vi "MODBUS  SLAVE.vi"() -> (3 "values to write":u16[](array[numeric]) caption="待写入值")   [LabVIEW 2016]
uses:
  <vilib>/NI/Modbus Library/Data Model/Device Data Model.lvclass
  <vilib>/NI/Modbus Library/API/Wrapper/Create TCP Slave.vi
  <vilib>/NI/Modbus Library/API/Slave/Modbus Slave.lvclass
  <vilib>/NI/Modbus Library/API/Wrapper/API Main.lvlib
panel:
  out "运行周期":u16[](array[numeric])
  in  "write operation starting address":u16=100 caption="写操作起始地址"
  out "单仪器启动命令":u16[](array[numeric])
  out "系统启动命令":u16[](array[numeric])
  in  "停止":bool
  out "register values":u16[](array[numeric]) caption="寄存器值"
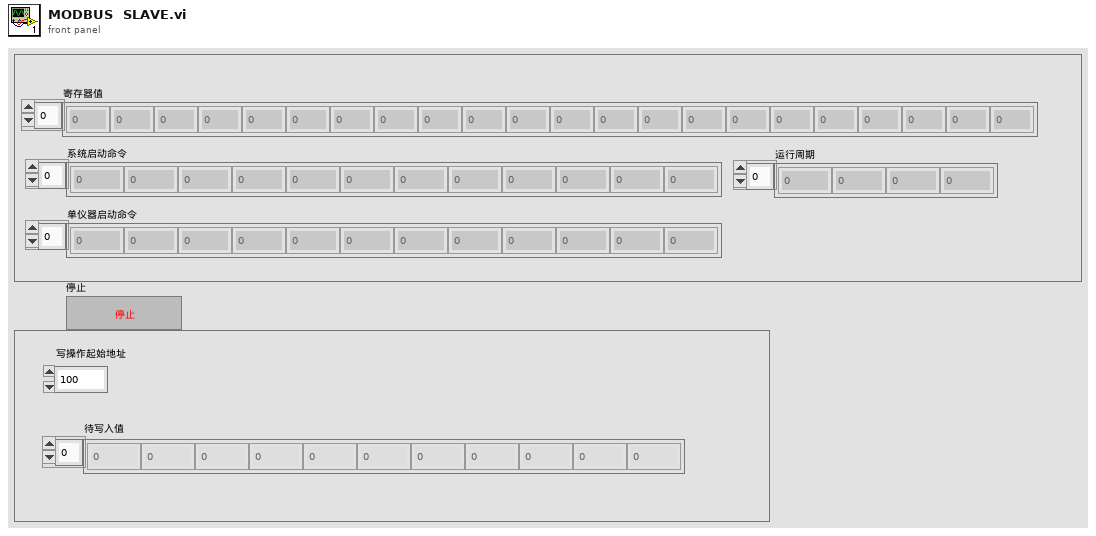
[diagram p1: front panel]
types:
  T1 = cluster{"测量模式":enum16{"水样测量", "标样核查", "零点核查", "跨度核查", "空白测试", "加标回收", "平行样", "校零", "校标"}}
  T2 = cluster{"站号":u16, "量程切换":enum32{"H", "L", "AUTO"}, "控制命令":enum16{"启动测量", "标样核查", "零点核查", "跨度核查", "空白测试", "平行样测试", "加标回收", "空白校准", "标样校准", "初始化（清洗）", "停止测试", "仪器重启", "校时", "模式设置", "测量间隔设置"}, "模式设置":enum16{"待机", "连续模式", "周期模式", "定点模式", "受控模式", "手动模式"}, "测量间隔":u16}
  T3 = cluster{"系统时间":timestamp, "工作状态":enum16{"空闲", "水样测试", "标样核查", "零点核查", "跨度核查", "空白测试", "平行样测试", "加标回收", "空白校准", "标样校准", "初始化（清洗）"}, "测量模式":enum16{"待机", "连续模式", "周期模式", "定点模式", "受控模式", "手动模式"}, "告警代码":enum16{"无告警", "缺试剂告警", "缺水样告警", "缺蒸馏水告警", "缺标液告警", "仪表漏液告警", "标定异常告警", "超量程告警", "加热异常", "低试剂预警", "超上限告警", "超下限告警", "仪表内部其他异常", "滴定异常告警", "电极异常告警", "量程切换告警", "参数设置告警", "PH电极电位异常", "电导率电极异常", "浊度光度异常", "溶解氧电极异常", "溶解氧光强异常", "温度异常告警", "PH异常告警", "溶解氧异常告警", "电导率异常告警", "浊度异常告警", "叶绿素异常告警", "藻密度异常告警", "蓝绿藻异常告警", "ORP异常告警", "氨氮异常告警", "清洁刷异常告警", "SD卡异常告警", "蓝牙异常告警", "Wifi异常告警", "流程异常告警"}, "故障代码":enum16{"无故障", "电机故障", "温度故障", "通讯故障", "滴定故障"}, "日志代码":u16, "软件版本":u16, "F0":sgl, "F1":sgl, "F2":sgl, "F3":sgl, "T":sgl, "H":sgl, "id":u16, "flowid":u16, "量程":u16, "总磷控温温度1":sgl, "营养盐控温温度2":sgl, "ADC":sgl}
  T4 = enum16{"空闲", "水样测试", "标样核查", "零点核查", "跨度核查", "空白测试", "平行样测试", "质控样", "空白校准", "标样校准", "加标回收"}
  T5 = enum16{"空闲", "水样测试", "标样核查", "零点核查", "跨度核查", "空白测试", "平行样测试", "加标回收", "空白校准", "标样校准", "初始化（清洗）"}
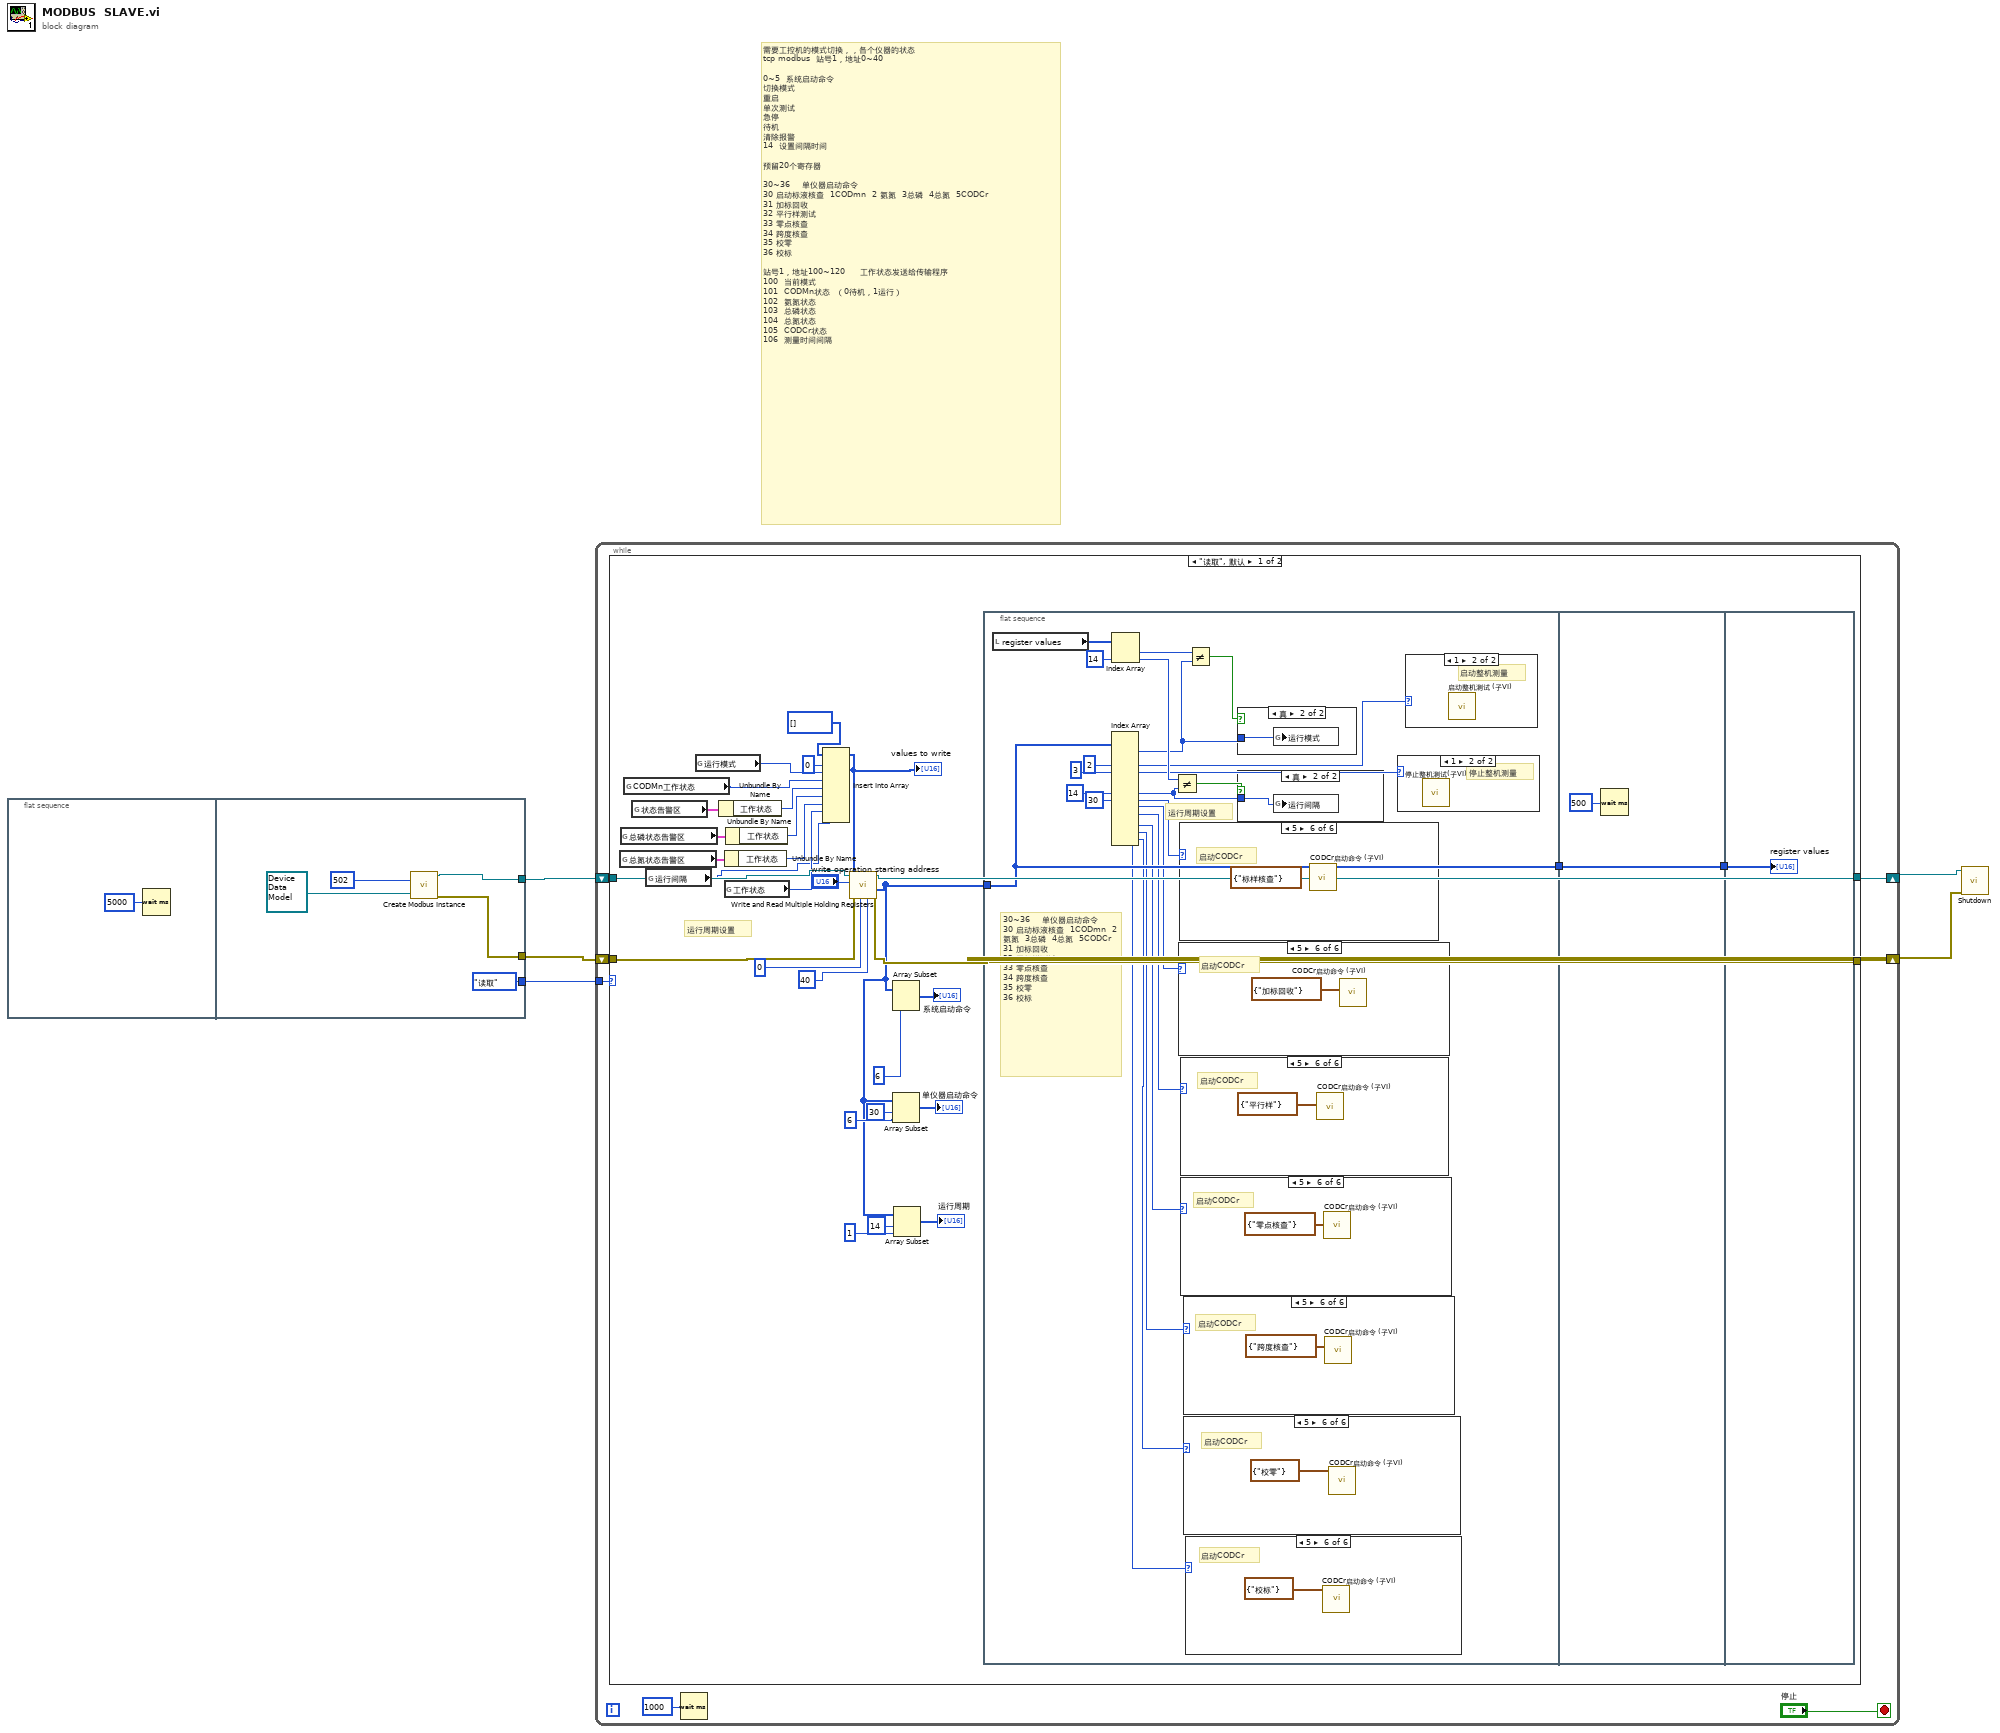
[diagram p0: block diagram]
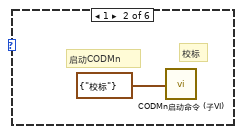
[diagram p3: hidden frame]
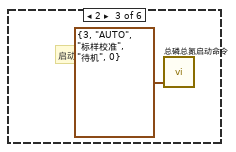
[diagram p4: hidden frame]
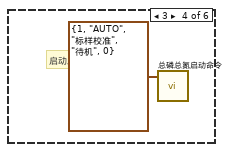
[diagram p5: hidden frame]
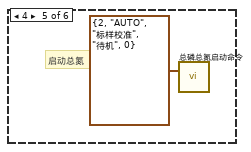
[diagram p6: hidden frame]
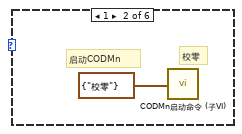
[diagram p8: hidden frame]
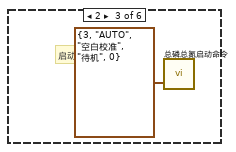
[diagram p9: hidden frame]
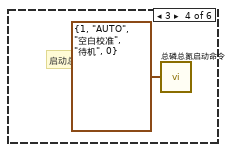
[diagram p10: hidden frame]
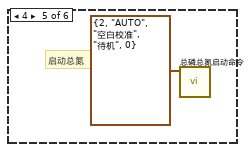
[diagram p11: hidden frame]
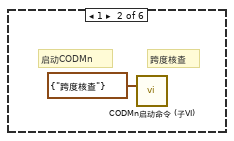
[diagram p13: hidden frame]
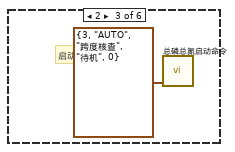
[diagram p14: hidden frame]
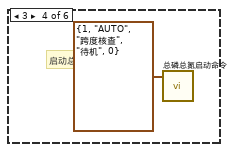
[diagram p15: hidden frame]
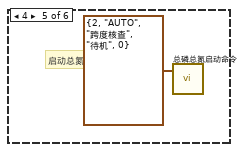
[diagram p16: hidden frame]
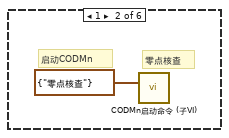
[diagram p18: hidden frame]
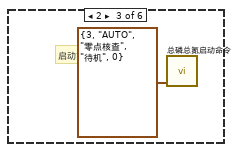
[diagram p19: hidden frame]
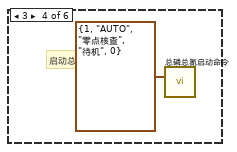
[diagram p20: hidden frame]
diagram:
  # "需要工控机的模式切换，，各个仪器的状态\ntcp modbus  站号1，地址0~40\n\n0~5  系统启动命令\n切换模式\n重启\n单次测试\n急停\n待机\n清除报警\n14  设置间隔时间\n\n预留20个寄存器\n\n30~36    单仪器启动命令\n30 启动标液核查  1CODmn  2 氨氮  3总磷  4总氮  5CODCr\n31 加标回收\n32 平行样测试\n33 零点核查\n34 跨度核查\n35 校零\n36 校标\n\n站号1，地址100~120     工作状态发送给传输程序\n100  当前模式\n101  CODMn状态  （0待机，1运行）\n102  氨氮状态\n103  总磷状态\n104  总氮状态\n105  CODCr状态\n106  测量时间间隔"
  n1 = flat-sequence {
    tunnel: [enum16{"读取", "写入"}."读取"] -> w5
    tunnel: [w9] -> w4
    tunnel: [w8] -> w3
    frame #0 {
      n2 = Wait (ms)(milliseconds to wait=u32 5000 ("等待时间（毫秒）")) -> ()  [unwired: 1 out]
    }
    frame #1 {
      n3 = call-poly <vilib>:"Create Modbus Instance.vi"("device data model"=refnum<class "Device Data Model.lvclass"> refnum, "port (502)"=u16 502) -> ("error out"=w8:errorcluster, "TCP slave instance"=w9:refnum<class "Modbus Slave.lvclass">)  [unwired: 8 in]
    }
  }
  n4 = while {
    shift-right: [w16] -> w2
    shift-left: w4 -> [w18]
    shift-right: [w12] -> w1
    shift-left: w3 -> [w17]
    tunnel: w5 -> [w13]
    stop <- "停止" stop-if-true
    n5 = case shown="\"读取\", 默认" w13 {
      tunnel: w18 -> [w45 w113]
      tunnel: w17 -> [w44 w112]
      tunnel: [w40 w113] -> w16
      tunnel: [w41 w112] -> w12
      frame "读取", Default {
        # "运行周期设置"
        n6 = global read "VAR总磷总氮全局变量.vi" "总氮状态告警区"() -> (w24:T3)
        n7 = global read "VAR总磷总氮全局变量.vi" "总磷状态告警区"() -> (w26:T3)
        n8 = global read "COD测量模式全局.vi" "CODMn工作状态"() -> (w22:T4)
        n9 = global read "VAR氨氮全局变量.vi" "状态告警区"() -> (w28:T3)
        n10 = global read "系统设置全局变量.vi" "运行间隔"() -> (w19:i16)
        n11 = global read "系统设置全局变量.vi" "运行模式"() -> (w20:enum16{"维护模式", "常规模式", "应急模式", "质控模式"})
        n12 = Unbundle By Name(w28) -> ("工作状态"=w27:T5)
        n13 = Unbundle By Name(w24) -> ("工作状态"=w23:T5)
        n14 = global read "CODcr全局变量.vi" "工作状态"() -> (w21:T5)
        n15 = Unbundle By Name(w26) -> ("工作状态"=w25:T5)
        n16 = Insert Into Array(array=u16[] [] ("values to write"), index=0 ("索引"), new element #1=w20, new element #2=w22, new element #3=w27, new element #4=w25, new element #5=w23, new element #6=w21, new element #7=w19) -> (w36:u16[])
        "values to write" <- w36
        n17 = call-dynamic "Write and Read Multiple Holding Registers.vi"("read count"=u16 40 ("number of holding registers"), "read starting address"=u16 0 ("starting address"), "error in"=w44, "write values"=w36, "write starting address"="write operation starting address", "Modbus instance in"=w45) -> ("error out"=w41:errorcluster, "read values"=w31:u16[], "Modbus instance out"=w40:refnum<class "Modbus Slave.lvclass">)  [unwired: 3 in]
        n18 = Array Subset(array=w31, length=6 ("长度")) -> (→"系统启动命令":u16[])  [unwired: 1 in]
        n19 = Array Subset(array=w31, index=30 ("索引"), length=6 ("长度")) -> (→"单仪器启动命令":u16[])
        n20 = Array Subset(array=w31, index=14 ("索引"), length=1 ("长度")) -> (→"运行周期":u16[])
        n21 = flat-sequence {
          tunnel: w31 -> [w71]
          tunnel: [w71] -> w30
          tunnel: w30 -> [w109]
          tunnel: [w109] -> w29
          tunnel: w29 -> [w111]
          frame #0 {
            # "运行周期设置"
            # "30~36    单仪器启动命令\n30 启动标液核查  1CODmn  2 氨氮  3总磷  4总氮  5CODCr\n31 加标回收\n32 平行样测试\n33 零点核查\n34 跨度核查\n35 校零\n36 校标"
            n22 = local read "register values"() -> (w70:u16[])
            n23 = Index Array(array=w71, index #3=2 ("索引"), index #4=3 ("索引"), index #7=14 ("索引"), index #8=30 ("索引")) -> (element #1=w58:u16, element #3=w59:u16, element #4=w60:u16, element #7=w61:u16, element #8=w56:u16, element #9=w55:u16, element #10=w54:u16, element #11=w53:u16, element #12=w52:u16, element #13=w51:u16, element #14=w50:u16)  [unwired: 10 in, 3 out]
            n24 = Index Array(array=w70, index #2=14 ("索引")) -> (element #1=w69:u16, element #2=w66:u16)  [unwired: 1 in]
            n25 = Not Equal?(x=w66, y=w61) -> (x != y?=w65:bool)
            n26 = case shown="5" w55 {
              frame 0, Default {
              }
              frame 1 {
                # "加标回收"
                # "启动CODMn"
                n27 = call "CODMn启动命令 (子VI).vi"("启动测量模式"=T1 {"测量模式"=enum."加标回收"}) -> ()  [unwired: 11 in]
              }
              frame 2 {
                # "启动氨氮"
                n28 = call "总磷总氮启动命令.vi"("参数"=T2 {"站号"=3, "量程切换"=enum."AUTO", "控制命令"=enum."加标回收", "模式设置"=enum."待机", "测量间隔"=0}) -> ()  [unwired: 10 in, 1 out]
              }
              frame 3 {
                # "启动总磷"
                n29 = call "总磷总氮启动命令.vi"("参数"=T2 {"站号"=1, "量程切换"=enum."AUTO", "控制命令"=enum."加标回收", "模式设置"=enum."待机", "测量间隔"=0}) -> ()  [unwired: 10 in, 1 out]
              }
              frame 4 {
                # "启动总氮"
                n30 = call "总磷总氮启动命令.vi"("参数"=T2 {"站号"=2, "量程切换"=enum."AUTO", "控制命令"=enum."加标回收", "模式设置"=enum."待机", "测量间隔"=0}) -> ()  [unwired: 10 in, 1 out]
              }
              frame 5 {
                # "启动CODCr"
                n31 = call "CODCr启动命令 (子VI).vi"("启动测量模式"=T1 {"测量模式"=enum."加标回收"}) -> ()  [unwired: 11 in]
              }
            }
            n32 = case shown="5" w56 {
              frame 0, Default {
              }
              frame 1 {
                # "启动标液核查"
                # "启动CODMn"
                n33 = call "CODMn启动命令 (子VI).vi"("启动测量模式"=T1 {"测量模式"=enum."标样核查"}) -> ()  [unwired: 11 in]
              }
              frame 2 {
                # "启动氨氮"
                n34 = call "总磷总氮启动命令.vi"("参数"=T2 {"站号"=3, "量程切换"=enum."AUTO", "控制命令"=enum."标样核查", "模式设置"=enum."待机", "测量间隔"=0}) -> ()  [unwired: 10 in, 1 out]
              }
              frame 3 {
                # "启动总磷"
                n35 = call "总磷总氮启动命令.vi"("参数"=T2 {"站号"=1, "量程切换"=enum."AUTO", "控制命令"=enum."标样核查", "模式设置"=enum."待机", "测量间隔"=0}) -> ()  [unwired: 10 in, 1 out]
              }
              frame 4 {
                # "启动总氮"
                n36 = call "总磷总氮启动命令.vi"("参数"=T2 {"站号"=2, "量程切换"=enum."AUTO", "控制命令"=enum."标样核查", "模式设置"=enum."待机", "测量间隔"=0}) -> ()  [unwired: 10 in, 1 out]
              }
              frame 5 {
                # "启动CODCr"
                n37 = call "CODCr启动命令 (子VI).vi"("启动测量模式"=T1 {"测量模式"=enum."标样核查"}) -> ()  [unwired: 11 in]
              }
            }
            n38 = case shown="5" w54 {
              frame 0, Default {
              }
              frame 1 {
                # "平行样测试"
                # "启动CODMn"
                n39 = call "CODMn启动命令 (子VI).vi"("启动测量模式"=T1 {"测量模式"=enum."平行样"}) -> ()  [unwired: 11 in]
              }
              frame 2 {
                # "启动氨氮"
                n40 = call "总磷总氮启动命令.vi"("参数"=T2 {"站号"=3, "量程切换"=enum."AUTO", "控制命令"=enum."平行样测试", "模式设置"=enum."待机", "测量间隔"=0}) -> ()  [unwired: 10 in, 1 out]
              }
              frame 3 {
                # "启动总磷"
                n41 = call "总磷总氮启动命令.vi"("参数"=T2 {"站号"=1, "量程切换"=enum."AUTO", "控制命令"=enum."平行样测试", "模式设置"=enum."待机", "测量间隔"=0}) -> ()  [unwired: 10 in, 1 out]
              }
              frame 4 {
                # "启动总氮"
                n42 = call "总磷总氮启动命令.vi"("参数"=T2 {"站号"=2, "量程切换"=enum."AUTO", "控制命令"=enum."平行样测试", "模式设置"=enum."待机", "测量间隔"=0}) -> ()  [unwired: 10 in, 1 out]
              }
              frame 5 {
                # "启动CODCr"
                n43 = call "CODCr启动命令 (子VI).vi"("启动测量模式"=T1 {"测量模式"=enum."平行样"}) -> ()  [unwired: 11 in]
              }
            }
            n44 = case shown="5" w53 {
              frame 0, Default {
              }
              frame 1 {
                # "零点核查"
                # "启动CODMn"
                n45 = call "CODMn启动命令 (子VI).vi"("启动测量模式"=T1 {"测量模式"=enum."零点核查"}) -> ()  [unwired: 11 in]
              }
              frame 2 {
                # "启动氨氮"
                n46 = call "总磷总氮启动命令.vi"("参数"=T2 {"站号"=3, "量程切换"=enum."AUTO", "控制命令"=enum."零点核查", "模式设置"=enum."待机", "测量间隔"=0}) -> ()  [unwired: 10 in, 1 out]
              }
              frame 3 {
                # "启动总磷"
                n47 = call "总磷总氮启动命令.vi"("参数"=T2 {"站号"=1, "量程切换"=enum."AUTO", "控制命令"=enum."零点核查", "模式设置"=enum."待机", "测量间隔"=0}) -> ()  [unwired: 10 in, 1 out]
              }
              frame 4 {
                # "启动总氮"
                n48 = call "总磷总氮启动命令.vi"("参数"=T2 {"站号"=2, "量程切换"=enum."AUTO", "控制命令"=enum."零点核查", "模式设置"=enum."待机", "测量间隔"=0}) -> ()  [unwired: 10 in, 1 out]
              }
              frame 5 {
                # "启动CODCr"
                n49 = call "CODCr启动命令 (子VI).vi"("启动测量模式"=T1 {"测量模式"=enum."零点核查"}) -> ()  [unwired: 11 in]
              }
            }
            n50 = case shown="5" w52 {
              frame 0, Default {
              }
              frame 1 {
                # "跨度核查"
                # "启动CODMn"
                n51 = call "CODMn启动命令 (子VI).vi"("启动测量模式"=T1 {"测量模式"=enum."跨度核查"}) -> ()  [unwired: 11 in]
              }
              frame 2 {
                # "启动氨氮"
                n52 = call "总磷总氮启动命令.vi"("参数"=T2 {"站号"=3, "量程切换"=enum."AUTO", "控制命令"=enum."跨度核查", "模式设置"=enum."待机", "测量间隔"=0}) -> ()  [unwired: 10 in, 1 out]
              }
              frame 3 {
                # "启动总磷"
                n53 = call "总磷总氮启动命令.vi"("参数"=T2 {"站号"=1, "量程切换"=enum."AUTO", "控制命令"=enum."跨度核查", "模式设置"=enum."待机", "测量间隔"=0}) -> ()  [unwired: 10 in, 1 out]
              }
              frame 4 {
                # "启动总氮"
                n54 = call "总磷总氮启动命令.vi"("参数"=T2 {"站号"=2, "量程切换"=enum."AUTO", "控制命令"=enum."跨度核查", "模式设置"=enum."待机", "测量间隔"=0}) -> ()  [unwired: 10 in, 1 out]
              }
              frame 5 {
                # "启动CODCr"
                n55 = call "CODCr启动命令 (子VI).vi"("启动测量模式"=T1 {"测量模式"=enum."跨度核查"}) -> ()  [unwired: 11 in]
              }
            }
            n56 = case shown="5" w51 {
              frame 0, Default {
              }
              frame 1 {
                # "校零"
                # "启动CODMn"
                n57 = call "CODMn启动命令 (子VI).vi"("启动测量模式"=T1 {"测量模式"=enum."校零"}) -> ()  [unwired: 11 in]
              }
              frame 2 {
                # "启动氨氮"
                n58 = call "总磷总氮启动命令.vi"("参数"=T2 {"站号"=3, "量程切换"=enum."AUTO", "控制命令"=enum."空白校准", "模式设置"=enum."待机", "测量间隔"=0}) -> ()  [unwired: 10 in, 1 out]
              }
              frame 3 {
                # "启动总磷"
                n59 = call "总磷总氮启动命令.vi"("参数"=T2 {"站号"=1, "量程切换"=enum."AUTO", "控制命令"=enum."空白校准", "模式设置"=enum."待机", "测量间隔"=0}) -> ()  [unwired: 10 in, 1 out]
              }
              frame 4 {
                # "启动总氮"
                n60 = call "总磷总氮启动命令.vi"("参数"=T2 {"站号"=2, "量程切换"=enum."AUTO", "控制命令"=enum."空白校准", "模式设置"=enum."待机", "测量间隔"=0}) -> ()  [unwired: 10 in, 1 out]
              }
              frame 5 {
                # "启动CODCr"
                n61 = call "CODCr启动命令 (子VI).vi"("启动测量模式"=T1 {"测量模式"=enum."校零"}) -> ()  [unwired: 11 in]
              }
            }
            n62 = case shown="5" w50 {
              frame 0, Default {
              }
              frame 1 {
                # "校标"
                # "启动CODMn"
                n63 = call "CODMn启动命令 (子VI).vi"("启动测量模式"=T1 {"测量模式"=enum."校标"}) -> ()  [unwired: 11 in]
              }
              frame 2 {
                # "启动氨氮"
                n64 = call "总磷总氮启动命令.vi"("参数"=T2 {"站号"=3, "量程切换"=enum."AUTO", "控制命令"=enum."标样校准", "模式设置"=enum."待机", "测量间隔"=0}) -> ()  [unwired: 10 in, 1 out]
              }
              frame 3 {
                # "启动总磷"
                n65 = call "总磷总氮启动命令.vi"("参数"=T2 {"站号"=1, "量程切换"=enum."AUTO", "控制命令"=enum."标样校准", "模式设置"=enum."待机", "测量间隔"=0}) -> ()  [unwired: 10 in, 1 out]
              }
              frame 4 {
                # "启动总氮"
                n66 = call "总磷总氮启动命令.vi"("参数"=T2 {"站号"=2, "量程切换"=enum."AUTO", "控制命令"=enum."标样校准", "模式设置"=enum."待机", "测量间隔"=0}) -> ()  [unwired: 10 in, 1 out]
              }
              frame 5 {
                # "启动CODCr"
                n67 = call "CODCr启动命令 (子VI).vi"("启动测量模式"=T1 {"测量模式"=enum."校标"}) -> ()  [unwired: 11 in]
              }
            }
            n68 = Not Equal?(x=w69, y=w58) -> (x != y?=w68:bool)
            n69 = case shown="真" w68 {
              tunnel: w58 -> [_ w108]
              frame False {
              }
              frame True {
                n70 = global write "系统设置全局变量.vi" "运行模式"(w108) -> ()
              }
            }
            n71 = case shown="真" w65 {
              tunnel: w61 -> [_ w107]
              frame False {
              }
              frame True {
                n72 = global write "系统设置全局变量.vi" "运行间隔"(w107) -> ()
              }
            }
            n73 = case shown="1" w60 {
              frame 0, Default {
              }
              frame 1 {
                # "停止整机测量"
                n74 = call "停止整机测试(子VI).vi"() -> ()  [unwired: 12 in]
              }
            }
            n75 = case shown="1" w59 {
              frame 0, Default {
              }
              frame 1 {
                # "启动整机测量"
                n76 = call "启动整机测试 (子VI).vi"() -> ()  [unwired: 12 in]
              }
            }
          }
          frame #1 {
            n77 = Wait (ms)(milliseconds to wait=u32 500 ("等待时间（毫秒）")) -> ()  [unwired: 1 out]
          }
          frame #2 {
            "register values" <- w111
          }
        }
      }
      frame "写入" {
      }
    }
    n78 = Wait (ms)(milliseconds to wait=u32 1000 ("等待时间（毫秒）")) -> ()  [unwired: 1 out]
  }
  n79 = call-dynamic "Shutdown.vi"("error in"=w1, "Modbus slave in"=w2) -> ()  [unwired: 9 in, 1 out]
